vi "ADO Command Get Integer Parameter Value.vi"(8 "error in (no error)":errorcluster, 10 "Index":i32, 11 "ADODB.Parameters":refnum<k7>) -> (0 "error out":errorcluster, 2 "Integer":i32, 3 "ADODB.Parameters":refnum<k7>)   [LabVIEW 2013]
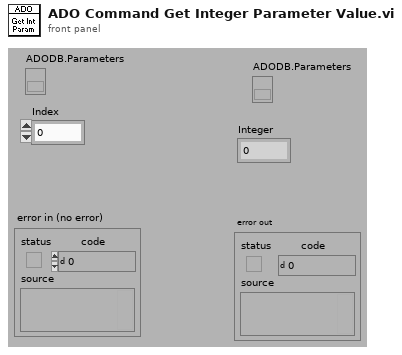
[diagram p1: front panel]
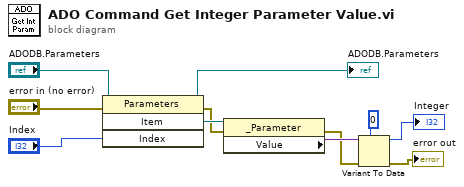
[diagram p0: block diagram]
diagram:
  n1 = invoke class="Parameters" method="Item"(reference="ADODB.Parameters", error in="error in (no error)", "Index"="Index") -> (reference out=→"ADODB.Parameters":refnum<k7>, error out=w10:errorcluster, "Item"=w11:refnum<k7>)  [unwired: 1 in, 1 out]
  n2 = property class="_Parameter"(reference=w11, error in=w10) -> (error out=w4:errorcluster, "Value"=w5:variant)  [unwired: 1 out]
  n3 = Variant To Data(error in=w4, type=0, Variant=w5) -> (data=→"Integer":i32, error out=→"error out":errorcluster)
